vi "PicoScope5000aSettings.vi"(0 "error in":errorcluster, 1 "Channel A Settings":T3={"Enabled"=FALSE, "Coupling"=1, "Range"=6, "Analogue Offset"=0.0, "Bandwidth Limit"=0} {"Bandwidth Limit" items=["Full", "20MHz"]; "Range" items=["10 mV", "20 mV", "50 mV", "100 mV", "200 mV", "500 mV", "1 V", "2 V", "5 V", "10 V", "20 V"]; "Coupling" items=["AC", "DC"]}, 2 "Port 0 Settings":T1={"Enabled"=FALSE, "Logic Level"=9830} {"Logic Level" items=["1.5V TTL"=9830, "2.5V CMOS"=16383]}, 3 "Channel B Settings":T3={"Enabled"=FALSE, "Coupling"=1, "Range"=6, "Analogue Offset"=0.0, "Bandwidth Limit"=0} {"Bandwidth Limit" items=["Full", "20MHz"]; "Range" items=["10 mV", "20 mV", "50 mV", "100 mV", "200 mV", "500 mV", "1 V", "2 V", "5 V", "10 V", "20 V"]; "Coupling" items=["AC", "DC"]}, 5 "handle in":i16, 9 "Device Info":T2, 11 "Trigger Settings":T4={"Trigger Enabled"=FALSE, "Trigger Source"=enum."Channel A", "Trigger Threshold (volts)"=0.0, "Trigger Direction"=2, "Trigger Delay (samples)"=0, "Auto Trigger Time (ms)"=1000} {"Trigger Direction" items=["Rising"=2, "Falling"=3]}, 12 "Channel C Settings":T3={"Enabled"=FALSE, "Coupling"=1, "Range"=6, "Analogue Offset"=0.0, "Bandwidth Limit"=0} {"Bandwidth Limit" items=["Full", "20MHz"]; "Range" items=["10 mV", "20 mV", "50 mV", "100 mV", "200 mV", "500 mV", "1 V", "2 V", "5 V", "10 V", "20 V"]; "Coupling" items=["AC", "DC"]}, 13 "Port 1 Settings":T1={"Enabled"=FALSE, "Logic Level"=9830} {"Logic Level" items=["1.5V TTL"=9830, "2.5V CMOS"=16383]}, 14 "Channel D Settings":T3={"Enabled"=FALSE, "Coupling"=1, "Range"=6, "Analogue Offset"=0.0, "Bandwidth Limit"=0} {"Bandwidth Limit" items=["Full", "20MHz"]; "Range" items=["10 mV", "20 mV", "50 mV", "100 mV", "200 mV", "500 mV", "1 V", "2 V", "5 V", "10 V", "20 V"]; "Coupling" items=["AC", "DC"]}, 15 "Max ADC value":i16) -> (4 "error out":errorcluster, 6 "handle out":i16, 8 "enabled array":i16[](array[numeric]))   [LabVIEW 2010]
doc: "This VI is used to set up the oscilloscope. The inputs are clusters for setting channel and simple trigger settings. Advanced triggers can be set up using PicoScope5000aAdvancedTriggerSettingsV2.vi"
uses:
  ps5000a.dll
  PicoScope5000aAnalogChannelSettings.ctl
  PicoScope5000aDigitalChannelSettings.ctl
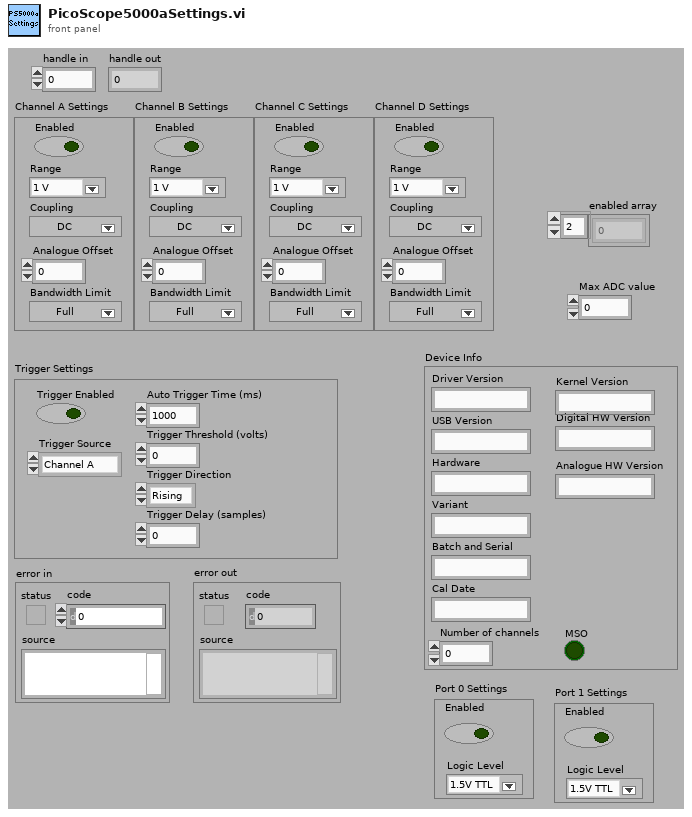
[diagram p1: front panel]
types:
  T1 = typedef "PicoScope5000aDigitalChannelSettings.ctl" = cluster{"Enabled":bool, "Logic Level":i16}
  T2 = cluster{"Driver Version":string, "USB Version":string, "Hardware":string, "Variant":string, "Batch and Serial":string, "Cal Date":string, "Kernel Version":string, "Digital HW Version":string, "Analogue HW Version":string, "MSO":bool, "Number of channels":i16}
  T3 = typedef "PicoScope5000aAnalogChannelSettings.ctl" = cluster{"Enabled":bool, "Coupling":i16, "Range":u16, "Analogue Offset":sgl, "Bandwidth Limit":u32}
  T4 = cluster{"Trigger Enabled":bool, "Trigger Source":enum16{"Channel A", "Channel B", "Channel C", "Channel D", "Ext."}, "Trigger Threshold (volts)":dbl, "Trigger Direction":u16, "Trigger Delay (samples)":u32, "Auto Trigger Time (ms)":i16}
  T5 = cluster{"status":bool, "code":u32, "source":string}
  T6 = enum16{"Channel A", "Channel B", "Channel C", "Channel D", "Ext."}
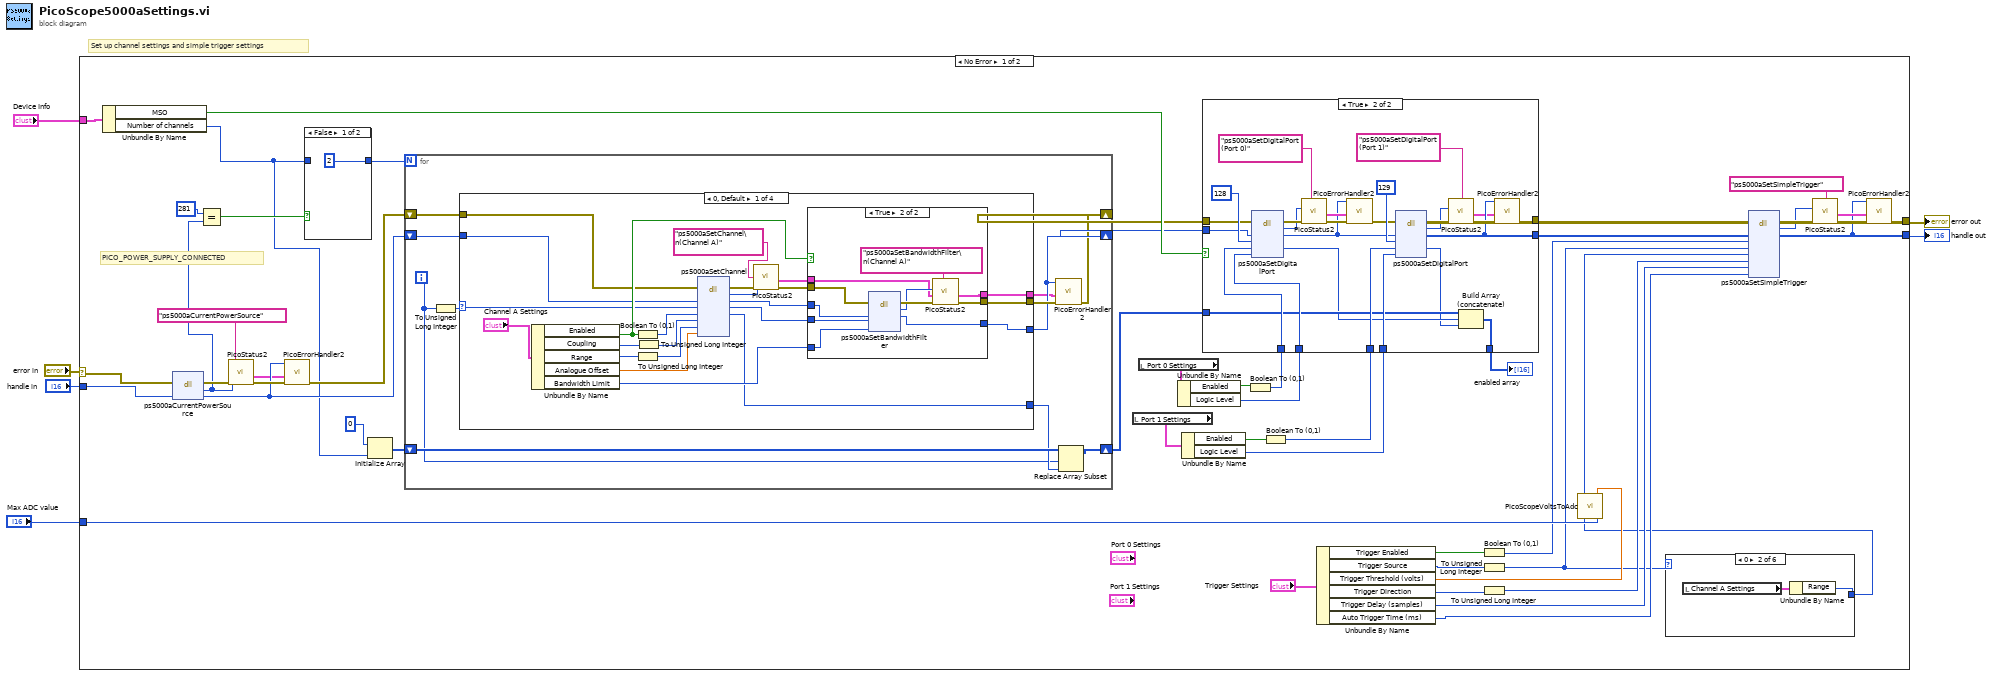
[diagram p0: block diagram]
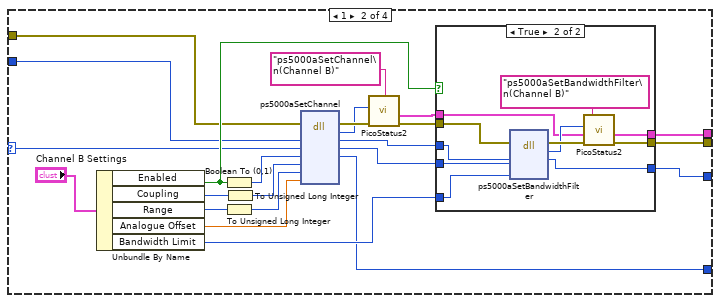
[diagram p4: hidden frame]
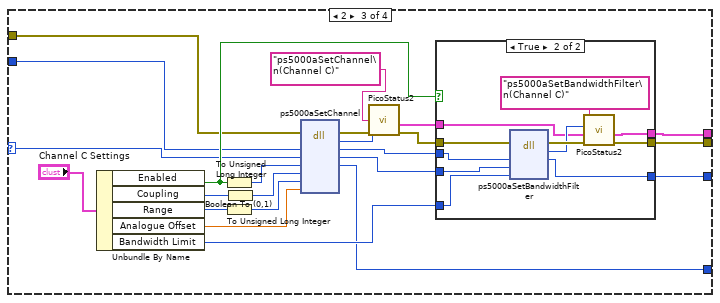
[diagram p6: hidden frame]
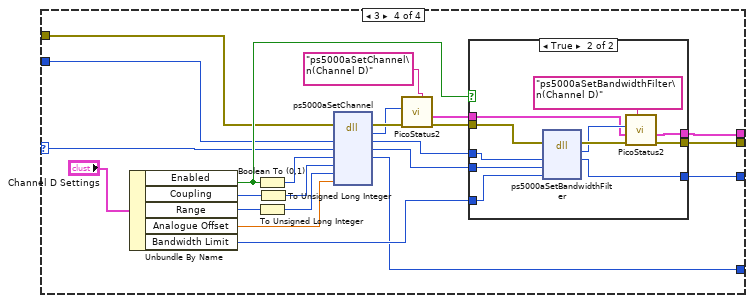
[diagram p8: hidden frame]
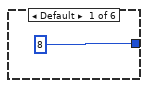
[diagram p11: hidden frame]
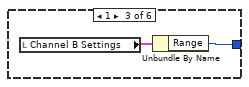
[diagram p12: hidden frame]
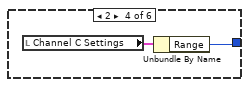
[diagram p13: hidden frame]
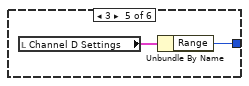
[diagram p14: hidden frame]
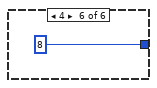
[diagram p15: hidden frame]
diagram:
  # "Set up channel settings and simple trigger settings"
  n1 = case shown="No Error" "error in" {
    selector: "error in" -> [w22 w259]
    tunnel: "handle in" -> [w21 w258]
    tunnel: [w7 w258] -> w4
    tunnel: [w8 w259] -> w3
    tunnel: "Device Info" -> [w44 _]
    tunnel: "Max ADC value" -> [w41 _]
    frame No Error {
      # "PICO_POWER_SUPPLY_CONNECTED"
      n2 = Unbundle By Name(w44) -> ("MSO"=w27:bool, "Number of channels"=w14:i16)
      n3 = dll-call lib="ps5000a.dll" fn="ps5000aCurrentPowerSource"(error in=w22, "handle"=w21) -> (error out=w47:errorcluster, "PICO_STATUS"=w45:u32, "handle"=w19:i16)  [unwired: 2 in, 1 out]
      n4 = Equal?(x=u32 281, y=w45) -> (x = y?=w17:bool)
      n5 = call "PicoStatus2.vi"("PICO source"="ps5000aCurrentPowerSource" ("source"), "Error in"=w47, "PICO STATUS"=w45) -> ("error out"=w20:errorcluster, "PICO_STATUS out"=w11:T5)  [unwired: 5 in]
      n6 = call "PicoErrorHandler2.vi"("error in (no error)"=w20, "PICO_STATUS in"=w11, "handle In"=w19) -> ("error out"=w18:errorcluster)  [unwired: 8 in]
      n7 = case shown="False" w17 {
        tunnel: [2 ("Number of channels") w59] -> w15
        tunnel: w14 -> [_ w59]
        frame False {
        }
        frame True {
        }
      }
      n8 = Initialize Array(i16 0 ("element"), w14) -> (w25:i16[])
      n9 = for {
        N: w15 -> [_]
        shift-right: [w68] -> w13
        shift-left: w25 -> [w70]
        shift-right: [w65] -> w24
        shift-left: w18 -> [w67]
        shift-right: [w63] -> w23
        shift-left: w19 -> [w66]
        i -> [w61]
        n10 = To Unsigned Long Integer(number=w61) -> (unsigned 32bit integer=w62:u32)
        n11 = case shown="0, Default" w62 {
          selector: w62 -> [w73 w110 w147 w184]
          tunnel: [w78 w116 w153 w190] -> w69
          tunnel: w67 -> [w77 w114 w151 w188]
          tunnel: w66 -> [w76 w113 w150 w187]
          tunnel: [w75 w112 w149 w186] -> w64
          tunnel: [w74 w111 w148 w185] -> w63
          tunnel: [w72 w108 w146 w183] -> w60
          frame 0, Default {
            n12 = Unbundle By Name("Channel A Settings") -> ("Enabled"=w82:bool, "Coupling"=w92:i16, "Range"=w93:u16, "Analogue Offset"=w90:sgl, "Bandwidth Limit"=w83:u32)
            n13 = Boolean To (0,1)(Boolean=w82) -> (0, 1=w85:i16)
            n14 = To Unsigned Long Integer(number=w93) -> (unsigned 32bit integer=w89:u32)
            n15 = To Unsigned Long Integer(number=w92) -> (unsigned 32bit integer=w91:u32)
            n16 = dll-call lib="ps5000a.dll" fn="ps5000aSetChannel" ("ps3000.dll:_ps3000_open_unit@0")(error in=w77, "handle"=w76, "channel"=w73, "enabled"=w85, "dc"=w91, "range"=w89, "analogueOffset"=w90) -> (error out=w88:errorcluster, "PICO_STATUS"=w87:u32, "handle"=w80:i16, "channel"=w79:u32, "enabled"=w78:i16)  [unwired: 5 in, 1 out]
            n17 = call "PicoStatus2.vi"("PICO source"="ps5000aSetChannel\n(Channel A)" ("source"), "Error in"=w88, "PICO STATUS"=w87) -> ("error out"=w81:errorcluster, "PICO_STATUS out"=w71:T5)  [unwired: 5 in]
            n18 = case shown="True" w82 {
              tunnel: w81 -> [w96 w104]
              tunnel: [w96 w103] -> w75
              tunnel: [w95 w102] -> w74
              tunnel: w79 -> [_ w101]
              tunnel: w80 -> [w95 w100]
              tunnel: w83 -> [_ w99]
              tunnel: [w94 w98] -> w72
              tunnel: w71 -> [w94 w97]
              frame False {
              }
              frame True {
                n19 = dll-call lib="ps5000a.dll" fn="ps5000aSetBandwidthFilter" ("ps3000.dll:_ps3000_open_unit@0")(error in=w104, "handle"=w100, "channel"=w101, "Bandwidth Limit"=w99) -> (error out=w106:errorcluster, "PICO_STATUS"=w105:u32, "handle"=w102:i16)  [unwired: 4 in, 1 out]
                n20 = call "PicoStatus2.vi"("PICO source"="ps5000aSetBandwidthFilter\n(Channel A)" ("source"), "Error in"=w106, "PICO_STATUS in"=w97, "PICO STATUS"=w105) -> ("error out"=w103:errorcluster, "PICO_STATUS out"=w98:T5)  [unwired: 4 in]
              }
            }
          }
          frame 1 {
            n21 = Unbundle By Name("Channel B Settings") -> ("Enabled"=w120:bool, "Coupling"=w129:i16, "Range"=w130:u16, "Analogue Offset"=w127:sgl, "Bandwidth Limit"=w121:u32)
            n22 = Boolean To (0,1)(Boolean=w120) -> (0, 1=w123:i16)
            n23 = To Unsigned Long Integer(number=w130) -> (unsigned 32bit integer=w126:u32)
            n24 = To Unsigned Long Integer(number=w129) -> (unsigned 32bit integer=w128:u32)
            n25 = dll-call lib="ps5000a.dll" fn="ps5000aSetChannel" ("ps3000.dll:_ps3000_open_unit@0")(error in=w114, "handle"=w113, "channel"=w110, "enabled"=w123, "dc"=w128, "range"=w126, "analogueOffset"=w127) -> (error out=w125:errorcluster, "PICO_STATUS"=w124:u32, "handle"=w118:i16, "channel"=w117:u32, "enabled"=w116:i16)  [unwired: 5 in, 1 out]
            n26 = call "PicoStatus2.vi"("PICO source"="ps5000aSetChannel\n(Channel B)" ("source"), "Error in"=w125, "PICO STATUS"=w124) -> ("error out"=w119:errorcluster, "PICO_STATUS out"=w109:T5)  [unwired: 5 in]
            n27 = case shown="True" w120 {
              tunnel: w119 -> [w133 w141]
              tunnel: [w133 w140] -> w112
              tunnel: [w132 w139] -> w111
              tunnel: w117 -> [_ w138]
              tunnel: w118 -> [w132 w137]
              tunnel: w121 -> [_ w136]
              tunnel: w109 -> [w131 w135]
              tunnel: [w131 w134] -> w108
              frame False {
              }
              frame True {
                n28 = dll-call lib="ps5000a.dll" fn="ps5000aSetBandwidthFilter" ("ps3000.dll:_ps3000_open_unit@0")(error in=w141, "handle"=w137, "channel"=w138, "Bandwidth Limit"=w136) -> (error out=w143:errorcluster, "PICO_STATUS"=w142:u32, "handle"=w139:i16)  [unwired: 4 in, 1 out]
                n29 = call "PicoStatus2.vi"("PICO source"="ps5000aSetBandwidthFilter\n(Channel B)" ("source"), "Error in"=w143, "PICO_STATUS in"=w135, "PICO STATUS"=w142) -> ("error out"=w140:errorcluster, "PICO_STATUS out"=w134:T5)  [unwired: 4 in]
              }
            }
          }
          frame 2 {
            n30 = Unbundle By Name("Channel C Settings") -> ("Enabled"=w157:bool, "Coupling"=w166:i16, "Range"=w167:u16, "Analogue Offset"=w164:sgl, "Bandwidth Limit"=w158:u32)
            n31 = Boolean To (0,1)(Boolean=w157) -> (0, 1=w160:i16)
            n32 = To Unsigned Long Integer(number=w167) -> (unsigned 32bit integer=w163:u32)
            n33 = To Unsigned Long Integer(number=w166) -> (unsigned 32bit integer=w165:u32)
            n34 = dll-call lib="ps5000a.dll" fn="ps5000aSetChannel" ("ps3000.dll:_ps3000_open_unit@0")(error in=w151, "handle"=w150, "channel"=w147, "enabled"=w160, "dc"=w165, "range"=w163, "analogueOffset"=w164) -> (error out=w162:errorcluster, "PICO_STATUS"=w161:u32, "handle"=w155:i16, "channel"=w154:u32, "enabled"=w153:i16)  [unwired: 5 in, 1 out]
            n35 = call "PicoStatus2.vi"("PICO source"="ps5000aSetChannel\n(Channel C)" ("source"), "Error in"=w162, "PICO STATUS"=w161) -> ("error out"=w156:errorcluster, "PICO_STATUS out"=w145:T5)  [unwired: 5 in]
            n36 = case shown="True" w157 {
              tunnel: w156 -> [w170 w178]
              tunnel: [w170 w177] -> w149
              tunnel: [w169 w176] -> w148
              tunnel: w154 -> [_ w175]
              tunnel: w155 -> [w169 w174]
              tunnel: w158 -> [_ w173]
              tunnel: [w168 w172] -> w146
              tunnel: w145 -> [w168 w171]
              frame False {
              }
              frame True {
                n37 = dll-call lib="ps5000a.dll" fn="ps5000aSetBandwidthFilter" ("ps3000.dll:_ps3000_open_unit@0")(error in=w178, "handle"=w174, "channel"=w175, "Bandwidth Limit"=w173) -> (error out=w180:errorcluster, "PICO_STATUS"=w179:u32, "handle"=w176:i16)  [unwired: 4 in, 1 out]
                n38 = call "PicoStatus2.vi"("PICO source"="ps5000aSetBandwidthFilter\n(Channel C)" ("source"), "Error in"=w180, "PICO_STATUS in"=w171, "PICO STATUS"=w179) -> ("error out"=w177:errorcluster, "PICO_STATUS out"=w172:T5)  [unwired: 4 in]
              }
            }
          }
          frame 3 {
            n39 = Unbundle By Name("Channel D Settings") -> ("Enabled"=w194:bool, "Coupling"=w203:i16, "Range"=w204:u16, "Analogue Offset"=w201:sgl, "Bandwidth Limit"=w195:u32)
            n40 = Boolean To (0,1)(Boolean=w194) -> (0, 1=w197:i16)
            n41 = To Unsigned Long Integer(number=w204) -> (unsigned 32bit integer=w200:u32)
            n42 = To Unsigned Long Integer(number=w203) -> (unsigned 32bit integer=w202:u32)
            n43 = dll-call lib="ps5000a.dll" fn="ps5000aSetChannel" ("ps3000.dll:_ps3000_open_unit@0")(error in=w188, "handle"=w187, "channel"=w184, "enabled"=w197, "dc"=w202, "range"=w200, "analogueOffset"=w201) -> (error out=w199:errorcluster, "PICO_STATUS"=w198:u32, "handle"=w192:i16, "channel"=w191:u32, "enabled"=w190:i16)  [unwired: 5 in, 1 out]
            n44 = call "PicoStatus2.vi"("PICO source"="ps5000aSetChannel\n(Channel D)" ("source"), "Error in"=w199, "PICO STATUS"=w198) -> ("error out"=w193:errorcluster, "PICO_STATUS out"=w182:T5)  [unwired: 5 in]
            n45 = case shown="True" w194 {
              tunnel: w193 -> [w207 w215]
              tunnel: [w207 w214] -> w186
              tunnel: [w206 w213] -> w185
              tunnel: w191 -> [_ w212]
              tunnel: w192 -> [w206 w211]
              tunnel: w195 -> [_ w210]
              tunnel: [w205 w209] -> w183
              tunnel: w182 -> [w205 w208]
              frame False {
              }
              frame True {
                n46 = dll-call lib="ps5000a.dll" fn="ps5000aSetBandwidthFilter" ("ps3000.dll:_ps3000_open_unit@0")(error in=w215, "handle"=w211, "channel"=w212, "Bandwidth Limit"=w210) -> (error out=w217:errorcluster, "PICO_STATUS"=w216:u32, "handle"=w213:i16)  [unwired: 4 in, 1 out]
                n47 = call "PicoStatus2.vi"("PICO source"="ps5000aSetBandwidthFilter\n(Channel D)" ("source"), "Error in"=w217, "PICO_STATUS in"=w208, "PICO STATUS"=w216) -> ("error out"=w214:errorcluster, "PICO_STATUS out"=w209:T5)  [unwired: 4 in]
              }
            }
          }
        }
        n48 = call "PicoErrorHandler2.vi"("error in (no error)"=w64, "PICO_STATUS in"=w60, "handle In"=w63) -> ("error out"=w65:errorcluster)  [unwired: 8 in]
        n49 = Replace Array Subset(array=w70, new element=w69, index=w61) -> (w68:i16[])
      }
      n50 = local read "Port 1 Settings"() -> (w37:T1)
      n51 = local read "Port 0 Settings"() -> (w38:T1)
      n52 = Unbundle By Name(w38) -> ("Enabled"=w36:bool, "Logic Level"=w34:i16)
      n53 = Unbundle By Name(w37) -> ("Enabled"=w33:bool, "Logic Level"=w31:i16)
      n54 = Boolean To (0,1)(Boolean=w36) -> (0, 1=w35:i16)
      n55 = Boolean To (0,1)(Boolean=w33) -> (0, 1=w32:i16)
      n56 = case shown="True" w27 {
        tunnel: [w221 w224] -> w30
        tunnel: w35 -> [_ w239]
        tunnel: w34 -> [_ w238]
        tunnel: w32 -> [_ w237]
        tunnel: w31 -> [_ w236]
        tunnel: w24 -> [w221 w235]
        tunnel: w23 -> [w220 w234]
        tunnel: [w220 w223] -> w29
        tunnel: w13 -> [w219 w233]
        tunnel: [w219 w230] -> w12
        frame False {
        }
        frame True {
          n57 = dll-call lib="PS5000a.dll" fn="ps5000aSetDigitalPort"(error in=w235, "handle"=w234, "port"=u32 128, "enabled"=w239, "logicLevel"=w238) -> (error out=w247:errorcluster, "PICO_STATUS"=w244:u32, "handle"=w227:i16, "enabled"=w232:i16)  [unwired: 4 in, 1 out]
          n58 = call "PicoStatus2.vi"("PICO source"="ps5000aSetDigitalPort (Port 0)" ("source"), "Error in"=w247, "PICO STATUS"=w244) -> ("error out"=w229:errorcluster, "PICO_STATUS out"=w228:T5)  [unwired: 5 in]
          n59 = call "PicoErrorHandler2.vi"("error in (no error)"=w229, "PICO_STATUS in"=w228, "handle In"=w227) -> ("error out"=w226:errorcluster)  [unwired: 8 in]
          n60 = dll-call lib="PS5000a.dll" fn="ps5000aSetDigitalPort"(error in=w226, "handle"=w227, "port"=u32 129, "enabled"=w237, "logicLevel"=w236) -> (error out=w243:errorcluster, "PICO_STATUS"=w242:u32, "handle"=w223:i16, "enabled"=w231:i16)  [unwired: 4 in, 1 out]
          n61 = call "PicoStatus2.vi"("PICO source"="ps5000aSetDigitalPort (Port 1)" ("source"), "Error in"=w243, "PICO STATUS"=w242) -> ("error out"=w225:errorcluster, "PICO_STATUS out"=w222:T5)  [unwired: 5 in]
          n62 = Build Array (concatenate)(w233, w232, w231) -> (w230:i16[])
          n63 = call "PicoErrorHandler2.vi"("error in (no error)"=w225, "PICO_STATUS in"=w222, "handle In"=w223) -> ("error out"=w224:errorcluster)  [unwired: 8 in]
        }
      }
      "enabled array" <- w12
      n64 = Unbundle By Name("Trigger Settings") -> ("Trigger Enabled"=w52:bool, "Trigger Source"=w53:T6, "Trigger Threshold (volts)"=w42:dbl, "Trigger Direction"=w55:u16, "Trigger Delay (samples)"=w54:u32, "Auto Trigger Time (ms)"=w40:i16)
      n65 = Boolean To (0,1)(Boolean=w52) -> (0, 1=w28:i16)
      n66 = To Unsigned Long Integer(number=w53) -> (unsigned 32bit integer=w39:u32)
      n67 = To Unsigned Long Integer(number=w55) -> (unsigned 32bit integer=w57:u32)
      n68 = case shown="0" w39 {
        tunnel: [u16 8 ("Range") w249 w251 w253 w255 u16 8 ("Range")] -> w16
        frame Default {
        }
        frame 0 {
          n69 = local read "Channel A Settings"() -> (w250:T3)
          n70 = Unbundle By Name(w250) -> ("Range"=w249:u16)
        }
        frame 1 {
          n71 = local read "Channel B Settings"() -> (w252:T3)
          n72 = Unbundle By Name(w252) -> ("Range"=w251:u16)
        }
        frame 2 {
          n73 = local read "Channel C Settings"() -> (w254:T3)
          n74 = Unbundle By Name(w254) -> ("Range"=w253:u16)
        }
        frame 3 {
          n75 = local read "Channel D Settings"() -> (w256:T3)
          n76 = Unbundle By Name(w256) -> ("Range"=w255:u16)
        }
        frame 4 {
        }
      }
      n77 = call "PicoScopeVoltsToAdc.vi"("Max_adc"=w41, "Units"=w42, "Range Index"=w16) -> ("ADC count"=w43:i16)
      n78 = dll-call lib="ps5000a.dll" fn="ps5000aSetSimpleTrigger" ("ps3000.dll:_ps3000_open_unit@0")(error in=w30, "handle"=w29, "enable"=w28, "source"=w39, "threshold"=w43, "direction"=w57, "delay"=w54, "autoTrigger_ms"=w40) -> (error out=w50:errorcluster, "PICO_STATUS"=w51:u32, "handle"=w7:i16)  [unwired: 8 in, 1 out]
      n79 = call "PicoStatus2.vi"("PICO source"="ps5000aSetSimpleTrigger" ("source"), "Error in"=w50, "PICO STATUS"=w51) -> ("error out"=w10:errorcluster, "PICO_STATUS out"=w9:T5)  [unwired: 5 in]
      n80 = call "PicoErrorHandler2.vi"("error in (no error)"=w10, "PICO_STATUS in"=w9, "handle In"=w7) -> ("error out"=w8:errorcluster)  [unwired: 8 in]
    }
    frame Error {
    }
  }
  "handle out" <- w4
  "error out" <- w3
